vi "Packet_decode_Int64.vi"(9 "StartByte":i32, 11 "RawData":u8[](array[numeric])) -> (1 "NextByte":i32, 3 "Int64_Value":i64)   [LabVIEW 2019, in "PhotonVisionLib.lvlib"]
doc: "Decode (or strip out) a 64 bit integer value from the provided byte array. No conversion or decoding is actually done, the memory is just copied, and the value is cast to the correct type.\n\nInputs\n - RawData -- Array of bytes containing the data to be extracted.\n - StartByte -- The starting byte number (the first byte starts at 0)\n\nOutputs\n - INT64_Value -- Extracted 64 bit integer value.\n - NextByte -- The starting byte index for the next value (regardless of type)."
uses:
  PhotonVisionLib.lvlib
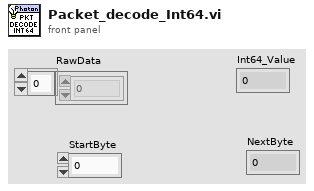
[diagram p1: front panel]
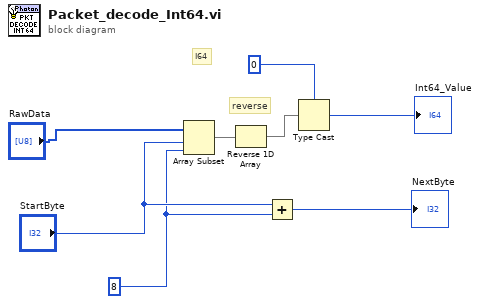
[diagram p0: block diagram]
diagram:
  w3 = 8 ("length")
  # "reverse"
  # "I64"
  n1 = Array Subset(array="RawData", index="StartByte", length=w3) -> (w2:u8[])
  n2 = Reverse 1D Array(array=w2) -> (reversed array=w1:u8[])
  n3 = Add(x="StartByte", y=w3) -> (x+y=→"NextByte":i32)
  n4 = Type Cast(type=i64 0, x=w1) -> (*(type *) &x=→"Int64_Value":i64)
